vi "Msgs Union.vi"(9 "Msgs 2":T1, 10 "Msgs 1":T1) -> (2 "Msgs Union":T1)   [LabVIEW 2020, in "jettl.lvlib" / "Actor.lvlib" / "Base Actor.lvclass"]
uses:
  Base Actor.lvclass
  Msg/Msg.lvclass
  Implemented Msgs.ctl
  Actor.lvlib
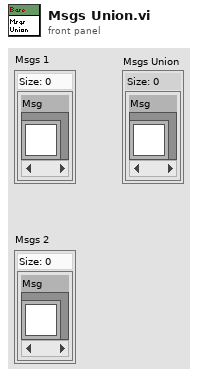
[diagram p1: front panel]
types:
  T1 = typedef "jettl.lvlib/Actor.lvlib/Implemented Msgs.ctl" = set{refnum<class "Msg.lvclass">}
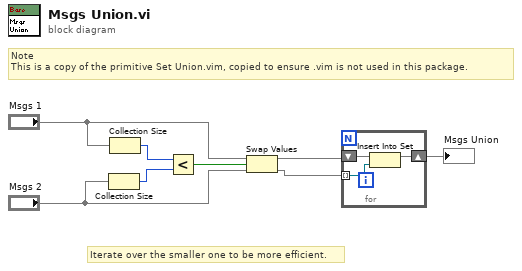
[diagram p0: block diagram]
diagram:
  # "Note\nThis is a copy of the primitive Set Union.vim, copied to ensure .vim is not used in this package."
  # "Iterate over the smaller one to be more efficient."
  n1 = Collection Size(1:"Msgs 2") -> (0:w7:i32)
  n2 = Collection Size(1:"Msgs 1") -> (0:w8:i32)
  n3 = Less?(x=w8, y=w7) -> (x < y?=w6:bool)
  n4 = Swap Values(12:"Msgs 1", 13:w6, 14:"Msgs 2") -> (1:w4:T1, 3:w5:T1)
  n5 = for {
    tunnel: w5 -> [w10] mode=indexing
    shift-right: [w9] -> w1
    shift-left: w4 -> [w11]
    n6 = Insert Into Set(10:w10, 11:w11) -> (3:w9:T1)  [unwired: 1 out]
  }
  "Msgs Union" <- w1
